vi "Memory.AnalogReplay.Selection.vi"(11 "memory":refnum<k21>="Replay Memory 0") -> (3 "memory":refnum<k21>="Replay Memory 0")   [LabVIEW 2015]
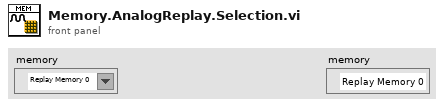
[diagram p1: front panel]
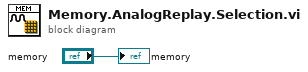
[diagram p0: block diagram]
diagram:
  "memory" <- "memory"
